vi "RS232_WR.vi"(8 "error in (no error)":errorcluster caption="错误输入（无错误）", 10 "CMD":string, 11 "VISA资源名称":refnum<visa-resource-name>) -> (0 "error out":errorcluster caption="错误输出", 2 "Out data":string[](array[string]), 3 "读取缓冲区":string)   [LabVIEW 2018]
panel:
  out "数组 2":string[](array[string])
  out "数组":string[](array[string])
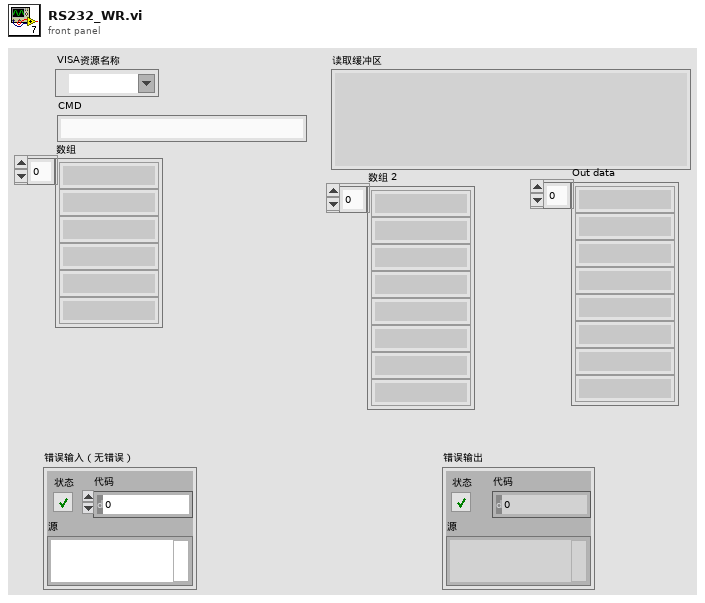
[diagram p1: front panel]
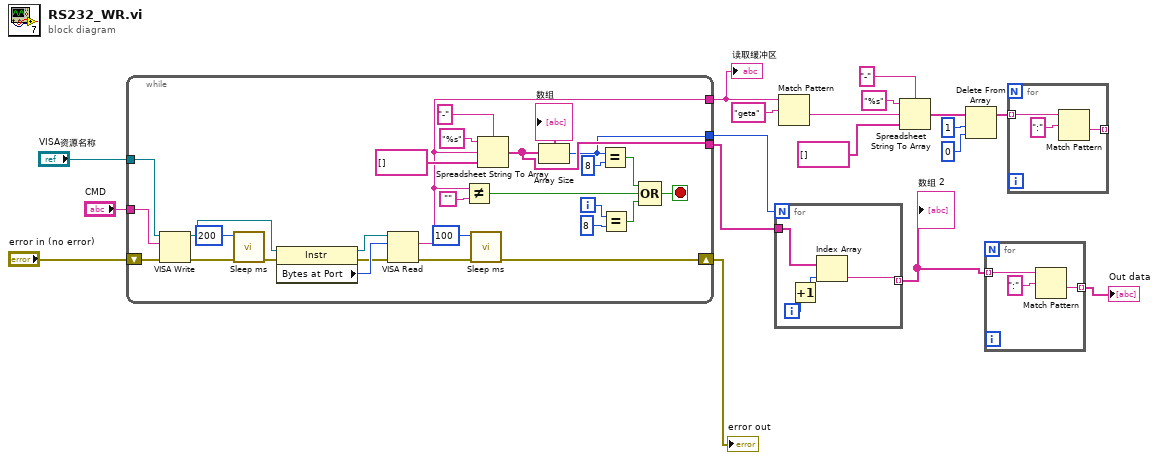
[diagram p0: block diagram]
diagram:
  n1 = while {
    tunnel: "VISA资源名称" -> [w44]
    tunnel: [w23] -> w6
    tunnel: "CMD" -> [w37]
    shift-right: [w27] -> w15
    shift-left: "error in (no error)" -> [w36]
    tunnel: [w20] -> w4
    tunnel: [w19] -> w3
    i -> [w33]
    stop <- w30 stop-if-true
    n2 = VISA Write(VISA resource name=w44, write buffer=w37, error in (no error)=w36) -> (VISA resource name out=w45:refnum<visa-resource-name>, error out=w43:errorcluster)  [unwired: 1 out]
    n3 = call "Sleep ms.vi"("error in (no error)"=w43, "等待时间（毫秒）"=u32 200) -> ("error out"=w42:errorcluster)  [unwired: 9 in]
    n4 = property class="Instr"(reference=w45, error in=w42) -> (reference out=w39:refnum<visa-resource-name>, error out=w38:errorcluster, "Bytes at Port"=w40:u32)
    n5 = VISA Read(VISA resource name=w39, byte count=w40, error in (no error)=w38) -> (read buffer=w23:string, error out=w28:errorcluster)  [unwired: 2 out]
    n6 = Not Equal?(x=w23, y="") -> (x != y?=w32:bool)
    n7 = call "Sleep ms.vi"("error in (no error)"=w28, "等待时间（毫秒）"=u32 100) -> ("error out"=w27:errorcluster)  [unwired: 9 in]
    n8 = Spreadsheet String To Array(delimiter (Tab)="-" ("分隔符(Tab)"), format string="%s" ("格式字符串"), spreadsheet string=w23, array type (2D Dbl)=string[] []) -> (array=w20:string[])
    "数组" <- w20
    n9 = Array Size(array=w20) -> (size(s)=w19:i32)
    n10 = Equal?(x=w19, y=8) -> (x = y?=w21:bool)
    n11 = Equal?(x=w33, y=8) -> (x = y?=w31:bool)
    n12 = Compound Arithmetic op=OR ("复合运算")(w21, w32, w31) -> (w30:bool)
  }
  "读取缓冲区" <- w6
  "error out" <- w15
  n13 = for {
    N: w3 -> [_]
    tunnel: w4 -> [w49]
    tunnel: [w47] -> w2 mode=indexing
    i -> [w48]
    n14 = Increment(x=w48) -> (x+1=w46:i32)
    n15 = Index Array(array=w49, index=w46) -> (element=w47:string)
  }
  "数组 2" <- w2
  n16 = Match Pattern(string=w6, regular expression="geta" ("正则表达式")) -> (after substring=w11:string)  [unwired: 1 in, 3 out]
  n17 = Spreadsheet String To Array(delimiter (Tab)="-" ("分隔符(Tab)"), format string="%s" ("格式字符串"), spreadsheet string=w11, array type (2D Dbl)=string[] []) -> (array=w12:string[])
  n18 = Delete From Array(array=w12, length=1 ("长度"), index=0 ("索引")) -> (array with subset deleted=w5:string[])  [unwired: 1 out]
  n19 = for {
    tunnel: w2 -> [w51] mode=indexing
    tunnel: [w50] -> w1 mode=indexing
    n20 = Match Pattern(string=w51, regular expression=":" ("正则表达式")) -> (after substring=w50:string)  [unwired: 1 in, 3 out]
  }
  "Out data" <- w1
  n21 = for {
    tunnel: w5 -> [w54] mode=indexing
    tunnel: [w53] -> _ mode=indexing
    n22 = Match Pattern(string=w54, regular expression=":" ("正则表达式")) -> (after substring=w53:string)  [unwired: 1 in, 3 out]
  }
